vi "Test_Config.vi"() -> (3 "All Passed":bool)   [LabVIEW 2021]
uses:
  a98184f2-8fd2-43de-8bb4-98a66dcb5e40.vi
  80b57f80-8d76-4516-95c7-d8f010efd1e0.vi
  85257279-96b8-465d-b682-86ad9ca409f4.vi
  dc8dce16-54c7-48e3-a8d0-ee2a6ed5b8ba.vi
  b43f0ab9-3a27-4143-a30c-0508d2798f1e.vi
  76b3366a-3206-4512-a529-652fa6d884ac.vi
  2d5518fb-c5ca-40ab-9de5-64a59f6f1d1f.vi
  2ff284ed-e038-49b9-b7c6-f7e4ced53d45.vi
  80cedbcb-86fa-476a-b55d-adc21445b371.vi
  4e733a6e-a8c1-4522-8606-2b13abc68f21.vi
  2655c138-ab8e-4111-a2df-5fe2dfe4a7c9.vi
  41d25b3f-7330-49a0-a764-42fdbbcff171.vi
  f7d9e632-003d-414d-bfce-bb79d7acb7ab.vi
  0279d870-c547-41fe-a729-ccd6f17232ba.vi
  8ff58d8c-39b3-443f-854e-0b9261e8d6a6.vi
  70d4e39b-dee4-4ea3-9cfd-b708fc97263a.vi
  a490dff2-e7e9-4792-baf0-702021434066.vi
  e326765a-9b9c-4b66-87f7-89ea6da7ec42.vi
  c037a717-6626-4282-85e0-497ccd3c4725.vi
  bc476a8b-c6ff-4744-88c1-a1946416cf06.vi
  3efe5734-2677-4856-90c7-08a3cd52a3b4.vi
  b62ae4c1-b65b-4156-9e59-aa89f562b7c2.vi
  d670cadd-57b7-44dd-9da6-c55518de0625.vi
  e85abf48-7778-4a54-96b8-6050ae3c274e.vi
  56efa82e-35ee-46c5-92d5-02654ef11c94.vi
  dab66c0f-6c3b-4909-9241-b858b76ef6f7.vi
  747298a2-2a9b-49bf-9d1b-76691c951ae0.vi
  29b0d965-e3aa-4d7c-908d-78c0fd6e1640.vi
  d4e3c187-ed36-4e66-b6bb-bd3ba352b96f.vi
  83e091ec-0c56-40c0-b4cc-2b8daf4164db.vi
  3d9b7528-4a5f-4daa-a7a8-b912a6b1f25e.vi
  f850aa45-a057-498a-96bd-8df103c2ec00.vi
  04663b24-a35a-4e7f-83d2-43bb6f822b82.vi
  9bed9d14-1784-4e91-a23c-442c56fd1ce7.vi
  cdbf88fd-1480-460b-834e-4cc60c3bbcb4.vi
  src/SubVIs/Quotes.vi
  src/SubVIs/Key.vi
  <vilib>/Utility/error.llb/Error Cluster From Error Code.vi
  src/Config.lvlib
panel:
  out "Tests":cluster{"Test":string, "Passed":bool}[](array[cluster])
  out "Text":string
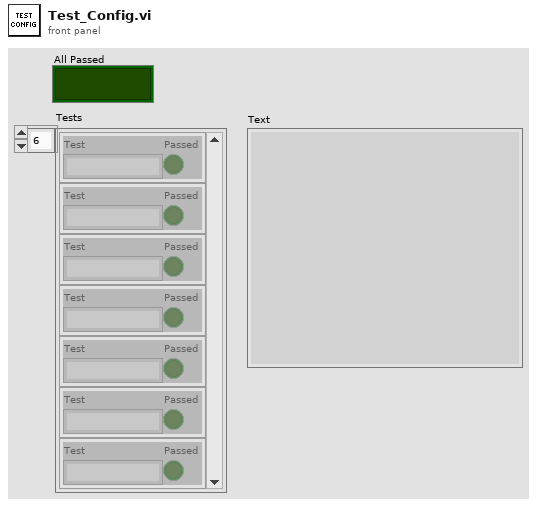
[diagram p1: front panel]
types:
  T1 = cluster{"Section":string, "Keys":cluster{"Key":string, "Value":string}[]}[]
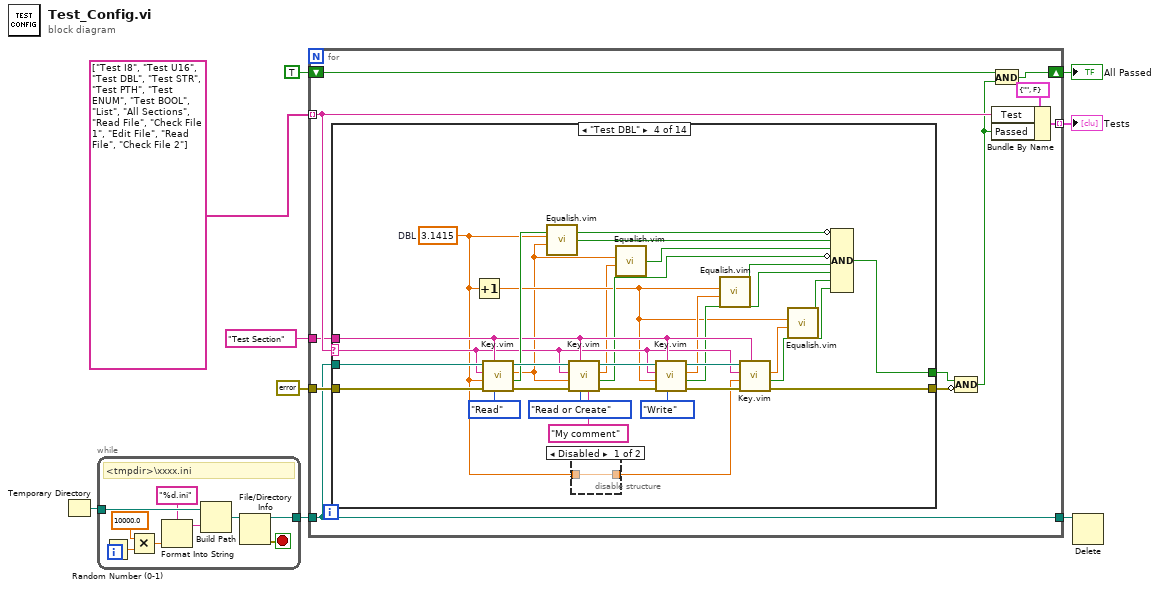
[diagram p0: block diagram]
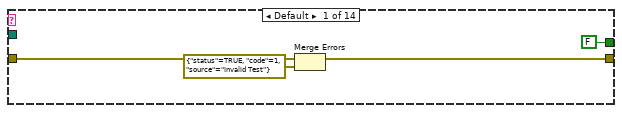
[diagram p2: hidden frame]
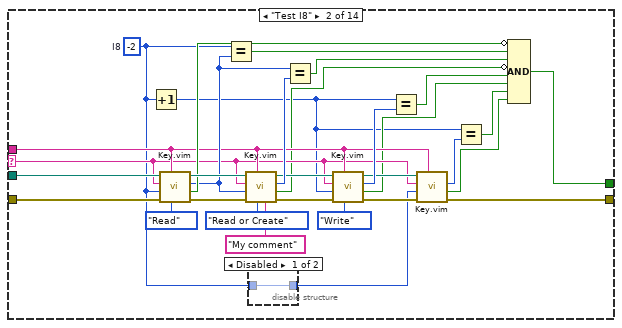
[diagram p3: hidden frame]
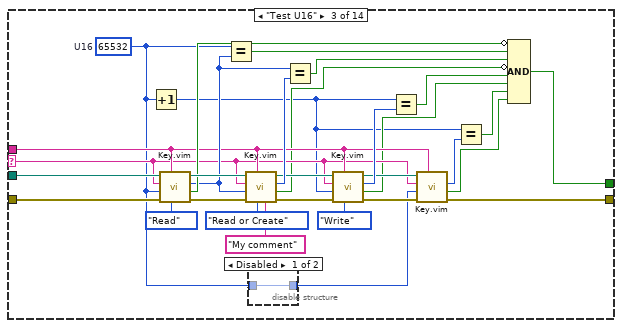
[diagram p5: hidden frame]
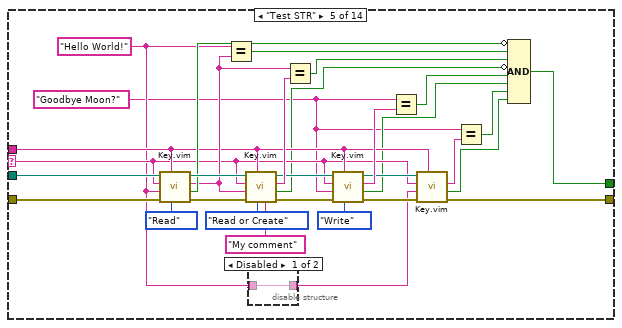
[diagram p8: hidden frame]
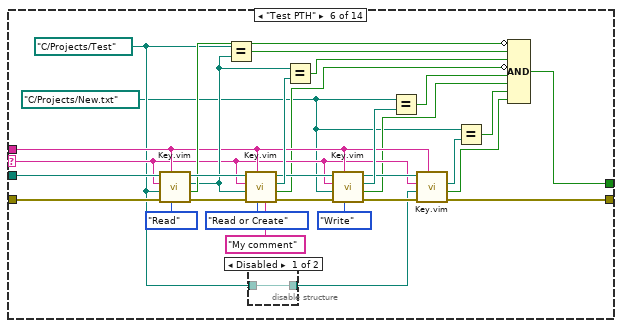
[diagram p10: hidden frame]
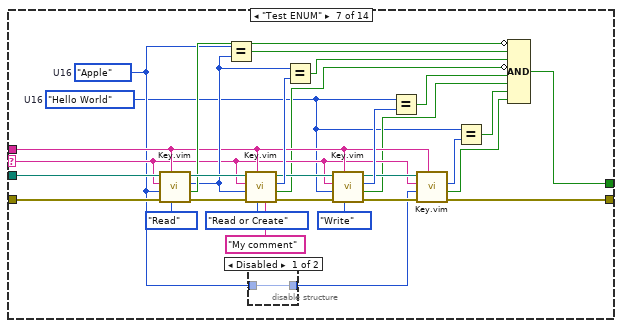
[diagram p12: hidden frame]
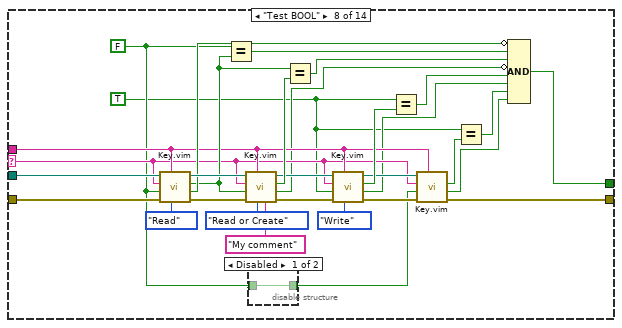
[diagram p14: hidden frame]
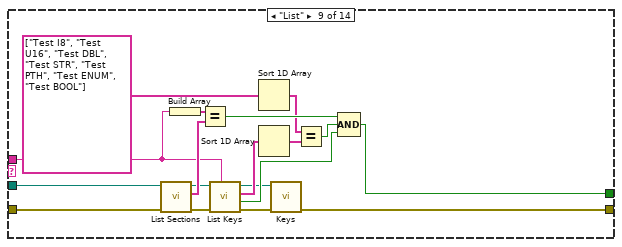
[diagram p16: hidden frame]
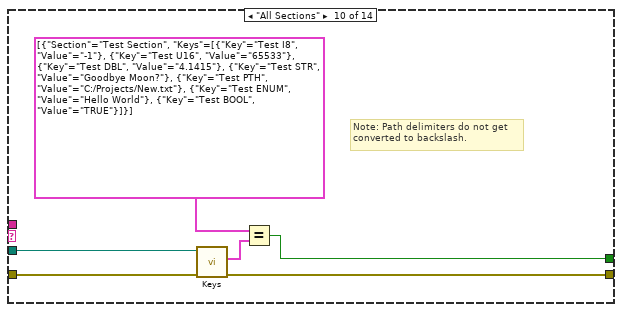
[diagram p17: hidden frame]
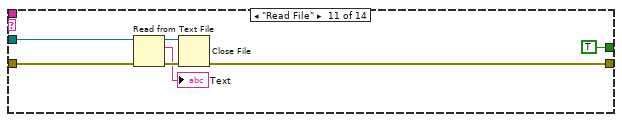
[diagram p18: hidden frame]
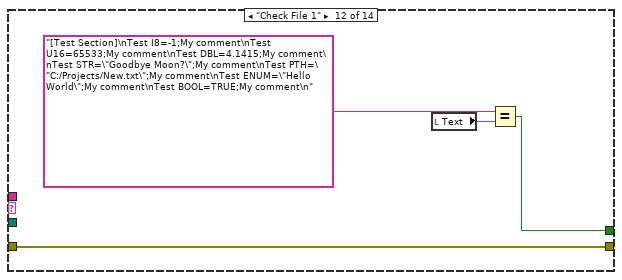
[diagram p19: hidden frame]
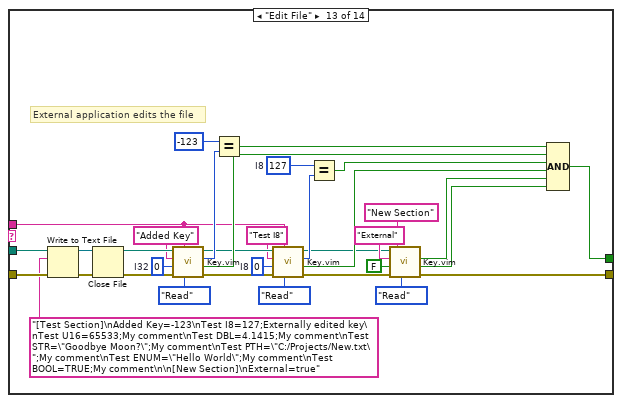
[diagram p20: hidden frame]
diagram:
  n1 = Temporary Directory() -> (w9:path)
  n2 = while {
    tunnel: w9 -> [w18]
    tunnel: [w10] -> w8
    stop <- w11 stop-if-true
    # "<tmpdir>\\xxxx.ini"
    n3 = Random Number (0-1)() -> (number: 0 to 1=w17:dbl)
    n4 = Multiply(x=10000.0 ("y"), y=w17) -> (x*y=w16:dbl)
    n5 = Format Into String(format string="%d.ini", w16) -> (resulting string=w13:string)  [unwired: 2 in, 1 out]
    n6 = Build Path(base path=w18, name or relative path=w13) -> (appended path=w12:path)
    n7 = File/Directory Info(path=w12) -> (path out=w10:path, error out=w11:errorcluster)  [unwired: 1 in, 5 out]
  }
  n8 = for {
    tunnel: w8 -> [w28]
    tunnel: errorcluster {"status"=FALSE, "code"=0, "source"=""} ("error out") -> [w29]
    tunnel: [w28] -> w6
    tunnel: string[] ["Test I8", "Test U16", "Test DBL", "Test STR", "Test PTH", "Test ENUM", "Test BOOL", "List", "All Sections", "Read File", "Check File 1", "Edit File", "Read File", "Check File 2"] ("array") -> [w24] mode=indexing
    tunnel: [w26] -> w5 mode=indexing
    shift-right: [w21] -> w2
    shift-left: TRUE -> [w22]
    tunnel: "Test Section" ("Section") -> [w19]
    n9 = case shown="\"Test DBL\"" w24 {
      selector: w24 -> [_ w44 w76 w114 w140 w172 w204 w236 _ _ _ _ _ _]
      tunnel: w29 -> [w33 w64 w96 w128 w160 w192 w224 w256 w275 w280 w286 w290 w324 w329]
      tunnel: w28 -> [_ w62 w94 w126 w158 w190 w222 w254 w274 w279 w285 _ w323 _]
      tunnel: [w32 w39 w71 w110 w135 w167 w200 w232 w260 w281 w284 w290 w293 w329] -> w23
      tunnel: w19 -> [_ w45 w77 w115 w141 w173 w205 w237 w269 _ _ _ w309 _]
      tunnel: [FALSE w34 w66 w108 w131 w163 w196 w228 w264 w277 TRUE w291 w306 w330] -> w25
      frame Default {
        n10 = Merge Errors(w33, errorcluster {"status"=TRUE, "code"=1, "source"="Invalid Test"} ("error in")) -> (w32:errorcluster)
      }
      frame "Test I8" {
        w40 = i8 -2  # I8
        n11 = Increment(x=w40) -> (x+1=w38:i8)
        n12 = call "Key.vim"("Operation (Read or Create)"=enum8{"Read or Create", "Read", "Write"}."Read", "Section"=w45, "error in (no error)"=w64, "Value"=w40, "Key"=w44, "Ini Path in"=w62) -> ("error out"=w60:errorcluster, "Found?"=w57:bool, "Value out"=w56:i8, "Ini Path out"=w59:path)  [unwired: 2 in]
        n13 = Equal?(x=w40, y=w56) -> (x = y?=w58:bool)
        n14 = call "Key.vim"("Comment (Create only)"="My comment", "Operation (Read or Create)"=enum8{"Read or Create", "Read", "Write"}."Read or Create", "Section"=w45, "error in (no error)"=w60, "Value"=w56, "Key"=w44, "Ini Path in"=w59) -> ("error out"=w51:errorcluster, "Found?"=w42:bool, "Value out"=w55:i8, "Ini Path out"=w50:path)  [unwired: 1 in]
        n15 = disable-structure shown="Disabled" {
          disable-tunnel: [w65 _] -> w41
          disable-tunnel: w40 -> [w65 _]
          frame Disabled {
          }
          frame Enabled {
          }
        }
        n16 = Equal?(x=w56, y=w55) -> (x = y?=w54:bool)
        n17 = call "Key.vim"("Operation (Read or Create)"=enum8{"Read or Create", "Read", "Write"}."Write", "Section"=w45, "error in (no error)"=w51, "Value"=w38, "Key"=w44, "Ini Path in"=w50) -> ("error out"=w47:errorcluster, "Found?"=w43:bool, "Value out"=w49:i8, "Ini Path out"=w46:path)  [unwired: 2 in]
        n18 = Equal?(x=w38, y=w49) -> (x = y?=w48:bool)
        n19 = call "Key.vim"("Section"=w45, "error in (no error)"=w47, "Value"=w41, "Key"=w44, "Ini Path in"=w46) -> ("error out"=w39:errorcluster, "Found?"=w35:bool, "Value out"=w37:i8)  [unwired: 3 in, 1 out]
        n20 = Equal?(x=w38, y=w37) -> (x = y?=w36:bool)
        n21 = Compound Arithmetic op=AND(invert w57, w58, w54, invert w42, w48, w43, w36, w35) -> (w34:bool)
      }
      frame "Test U16" {
        w72 = u16 65532  # U16
        n22 = Increment(x=w72) -> (x+1=w70:u16)
        n23 = call "Key.vim"("Operation (Read or Create)"=enum8{"Read or Create", "Read", "Write"}."Read", "Section"=w77, "error in (no error)"=w96, "Value"=w72, "Key"=w76, "Ini Path in"=w94) -> ("error out"=w92:errorcluster, "Found?"=w89:bool, "Value out"=w88:u16, "Ini Path out"=w91:path)  [unwired: 2 in]
        n24 = Equal?(x=w72, y=w88) -> (x = y?=w90:bool)
        n25 = call "Key.vim"("Comment (Create only)"="My comment", "Operation (Read or Create)"=enum8{"Read or Create", "Read", "Write"}."Read or Create", "Section"=w77, "error in (no error)"=w92, "Value"=w88, "Key"=w76, "Ini Path in"=w91) -> ("error out"=w83:errorcluster, "Found?"=w74:bool, "Value out"=w87:u16, "Ini Path out"=w82:path)  [unwired: 1 in]
        n26 = disable-structure shown="Disabled" {
          disable-tunnel: [w97 _] -> w73
          disable-tunnel: w72 -> [w97 _]
          frame Disabled {
          }
          frame Enabled {
          }
        }
        n27 = Equal?(x=w88, y=w87) -> (x = y?=w86:bool)
        n28 = call "Key.vim"("Operation (Read or Create)"=enum8{"Read or Create", "Read", "Write"}."Write", "Section"=w77, "error in (no error)"=w83, "Value"=w70, "Key"=w76, "Ini Path in"=w82) -> ("error out"=w79:errorcluster, "Found?"=w75:bool, "Value out"=w81:u16, "Ini Path out"=w78:path)  [unwired: 2 in]
        n29 = Equal?(x=w70, y=w81) -> (x = y?=w80:bool)
        n30 = call "Key.vim"("Section"=w77, "error in (no error)"=w79, "Value"=w73, "Key"=w76, "Ini Path in"=w78) -> ("error out"=w71:errorcluster, "Found?"=w67:bool, "Value out"=w69:u16)  [unwired: 3 in, 1 out]
        n31 = Equal?(x=w70, y=w69) -> (x = y?=w68:bool)
        n32 = Compound Arithmetic op=AND(invert w89, w90, w86, invert w74, w80, w75, w68, w67) -> (w66:bool)
      }
      frame "Test DBL" {
        w102 = 3.1415  # DBL
        n33 = Increment(x=w102) -> (x+1=w105:dbl)
        n34 = call "Key.vim"("Operation (Read or Create)"=enum8{"Read or Create", "Read", "Write"}."Read", "Section"=w115, "error in (no error)"=w128, "Value"=w102, "Key"=w114, "Ini Path in"=w126) -> ("error out"=w124:errorcluster, "Found?"=w122:bool, "Value out"=w100:dbl, "Ini Path out"=w123:path)  [unwired: 2 in]
        n35 = call "Equalish.vim"("First"=w102, "Second"=w100) -> ("Equal?"=w101:bool)  [unwired: 3 in]
        n36 = call "Key.vim"("Comment (Create only)"="My comment", "Operation (Read or Create)"=enum8{"Read or Create", "Read", "Write"}."Read or Create", "Section"=w115, "error in (no error)"=w124, "Value"=w100, "Key"=w114, "Ini Path in"=w123) -> ("error out"=w119:errorcluster, "Found?"=w112:bool, "Value out"=w99:dbl, "Ini Path out"=w118:path)  [unwired: 1 in]
        n37 = disable-structure shown="Disabled" {
          disable-tunnel: [w129 _] -> w111
          disable-tunnel: w102 -> [w129 _]
          frame Disabled {
          }
          frame Enabled {
          }
        }
        n38 = call "Equalish.vim"("First"=w100, "Second"=w99) -> ("Equal?"=w98:bool)  [unwired: 3 in]
        n39 = call "Key.vim"("Operation (Read or Create)"=enum8{"Read or Create", "Read", "Write"}."Write", "Section"=w115, "error in (no error)"=w119, "Value"=w105, "Key"=w114, "Ini Path in"=w118) -> ("error out"=w117:errorcluster, "Found?"=w113:bool, "Value out"=w107:dbl, "Ini Path out"=w116:path)  [unwired: 2 in]
        n40 = call "Equalish.vim"("First"=w105, "Second"=w107) -> ("Equal?"=w106:bool)  [unwired: 3 in]
        n41 = call "Key.vim"("Section"=w115, "error in (no error)"=w117, "Value"=w111, "Key"=w114, "Ini Path in"=w116) -> ("error out"=w110:errorcluster, "Found?"=w109:bool, "Value out"=w104:dbl)  [unwired: 3 in, 1 out]
        n42 = call "Equalish.vim"("First"=w105, "Second"=w104) -> ("Equal?"=w103:bool)  [unwired: 3 in]
        n43 = Compound Arithmetic op=AND(invert w122, w101, w98, invert w112, w106, w113, w103, w109) -> (w108:bool)
      }
      frame "Test STR" {
        w130 = "Goodbye Moon?"
        w136 = "Hello World!"
        n44 = call "Key.vim"("Operation (Read or Create)"=enum8{"Read or Create", "Read", "Write"}."Read", "Section"=w141, "error in (no error)"=w160, "Value"=w136, "Key"=w140, "Ini Path in"=w158) -> ("error out"=w156:errorcluster, "Found?"=w153:bool, "Value out"=w152:string, "Ini Path out"=w155:path)  [unwired: 2 in]
        n45 = Equal?(x=w136, y=w152) -> (x = y?=w154:bool)
        n46 = call "Key.vim"("Comment (Create only)"="My comment", "Operation (Read or Create)"=enum8{"Read or Create", "Read", "Write"}."Read or Create", "Section"=w141, "error in (no error)"=w156, "Value"=w152, "Key"=w140, "Ini Path in"=w155) -> ("error out"=w147:errorcluster, "Found?"=w138:bool, "Value out"=w151:string, "Ini Path out"=w146:path)  [unwired: 1 in]
        n47 = disable-structure shown="Disabled" {
          disable-tunnel: [w161 _] -> w137
          disable-tunnel: w136 -> [w161 _]
          frame Disabled {
          }
          frame Enabled {
          }
        }
        n48 = Equal?(x=w152, y=w151) -> (x = y?=w150:bool)
        n49 = call "Key.vim"("Operation (Read or Create)"=enum8{"Read or Create", "Read", "Write"}."Write", "Section"=w141, "error in (no error)"=w147, "Value"=w130, "Key"=w140, "Ini Path in"=w146) -> ("error out"=w143:errorcluster, "Found?"=w139:bool, "Value out"=w145:string, "Ini Path out"=w142:path)  [unwired: 2 in]
        n50 = Equal?(x=w130, y=w145) -> (x = y?=w144:bool)
        n51 = call "Key.vim"("Section"=w141, "error in (no error)"=w143, "Value"=w137, "Key"=w140, "Ini Path in"=w142) -> ("error out"=w135:errorcluster, "Found?"=w132:bool, "Value out"=w134:string)  [unwired: 3 in, 1 out]
        n52 = Equal?(x=w130, y=w134) -> (x = y?=w133:bool)
        n53 = Compound Arithmetic op=AND(invert w153, w154, w150, invert w138, w144, w139, w133, w132) -> (w131:bool)
      }
      frame "Test PTH" {
        w162 = path "C:/Projects/New.txt"
        w168 = path "C:/Projects/Test"
        n54 = call "Key.vim"("Operation (Read or Create)"=enum8{"Read or Create", "Read", "Write"}."Read", "Section"=w173, "error in (no error)"=w192, "Value"=w168, "Key"=w172, "Ini Path in"=w190) -> ("error out"=w188:errorcluster, "Found?"=w185:bool, "Value out"=w184:path, "Ini Path out"=w187:path)  [unwired: 2 in]
        n55 = Equal?(x=w168, y=w184) -> (x = y?=w186:bool)
        n56 = call "Key.vim"("Comment (Create only)"="My comment", "Operation (Read or Create)"=enum8{"Read or Create", "Read", "Write"}."Read or Create", "Section"=w173, "error in (no error)"=w188, "Value"=w184, "Key"=w172, "Ini Path in"=w187) -> ("error out"=w179:errorcluster, "Found?"=w170:bool, "Value out"=w183:path, "Ini Path out"=w178:path)  [unwired: 1 in]
        n57 = disable-structure shown="Disabled" {
          disable-tunnel: [w193 _] -> w169
          disable-tunnel: w168 -> [w193 _]
          frame Disabled {
          }
          frame Enabled {
          }
        }
        n58 = Equal?(x=w184, y=w183) -> (x = y?=w182:bool)
        n59 = call "Key.vim"("Operation (Read or Create)"=enum8{"Read or Create", "Read", "Write"}."Write", "Section"=w173, "error in (no error)"=w179, "Value"=w162, "Key"=w172, "Ini Path in"=w178) -> ("error out"=w175:errorcluster, "Found?"=w171:bool, "Value out"=w177:path, "Ini Path out"=w174:path)  [unwired: 2 in]
        n60 = Equal?(x=w162, y=w177) -> (x = y?=w176:bool)
        n61 = call "Key.vim"("Section"=w173, "error in (no error)"=w175, "Value"=w169, "Key"=w172, "Ini Path in"=w174) -> ("error out"=w167:errorcluster, "Found?"=w164:bool, "Value out"=w166:path)  [unwired: 3 in, 1 out]
        n62 = Equal?(x=w162, y=w166) -> (x = y?=w165:bool)
        n63 = Compound Arithmetic op=AND(invert w185, w186, w182, invert w170, w176, w171, w165, w164) -> (w163:bool)
      }
      frame "Test ENUM" {
        w194 = enum16{"Apple", "Hello World", "Item 3"}."Hello World"  # U16
        w195 = enum16{"Apple", "Hello World", "Item 3"}."Apple"  # U16
        n64 = call "Key.vim"("Operation (Read or Create)"=enum8{"Read or Create", "Read", "Write"}."Read", "Section"=w205, "error in (no error)"=w224, "Value"=w195, "Key"=w204, "Ini Path in"=w222) -> ("error out"=w220:errorcluster, "Found?"=w217:bool, "Value out"=w216:enum16{"Apple", "Hello World", "Item 3"}, "Ini Path out"=w219:path)  [unwired: 2 in]
        n65 = Equal?(x=w195, y=w216) -> (x = y?=w218:bool)
        n66 = call "Key.vim"("Comment (Create only)"="My comment", "Operation (Read or Create)"=enum8{"Read or Create", "Read", "Write"}."Read or Create", "Section"=w205, "error in (no error)"=w220, "Value"=w216, "Key"=w204, "Ini Path in"=w219) -> ("error out"=w211:errorcluster, "Found?"=w202:bool, "Value out"=w215:enum16{"Apple", "Hello World", "Item 3"}, "Ini Path out"=w210:path)  [unwired: 1 in]
        n67 = disable-structure shown="Disabled" {
          disable-tunnel: [w225 _] -> w201
          disable-tunnel: w195 -> [w225 _]
          frame Disabled {
          }
          frame Enabled {
          }
        }
        n68 = Equal?(x=w216, y=w215) -> (x = y?=w214:bool)
        n69 = call "Key.vim"("Operation (Read or Create)"=enum8{"Read or Create", "Read", "Write"}."Write", "Section"=w205, "error in (no error)"=w211, "Value"=w194, "Key"=w204, "Ini Path in"=w210) -> ("error out"=w207:errorcluster, "Found?"=w203:bool, "Value out"=w209:enum16{"Apple", "Hello World", "Item 3"}, "Ini Path out"=w206:path)  [unwired: 2 in]
        n70 = Equal?(x=w194, y=w209) -> (x = y?=w208:bool)
        n71 = call "Key.vim"("Section"=w205, "error in (no error)"=w207, "Value"=w201, "Key"=w204, "Ini Path in"=w206) -> ("error out"=w200:errorcluster, "Found?"=w197:bool, "Value out"=w199:enum16{"Apple", "Hello World", "Item 3"})  [unwired: 3 in, 1 out]
        n72 = Equal?(x=w194, y=w199) -> (x = y?=w198:bool)
        n73 = Compound Arithmetic op=AND(invert w217, w218, w214, invert w202, w208, w203, w198, w197) -> (w196:bool)
      }
      frame "Test BOOL" {
        w226 = TRUE
        w227 = FALSE
        n74 = call "Key.vim"("Operation (Read or Create)"=enum8{"Read or Create", "Read", "Write"}."Read", "Section"=w237, "error in (no error)"=w256, "Value"=w227, "Key"=w236, "Ini Path in"=w254) -> ("error out"=w252:errorcluster, "Found?"=w249:bool, "Value out"=w248:bool, "Ini Path out"=w251:path)  [unwired: 2 in]
        n75 = Equal?(x=w227, y=w248) -> (x = y?=w250:bool)
        n76 = call "Key.vim"("Comment (Create only)"="My comment", "Operation (Read or Create)"=enum8{"Read or Create", "Read", "Write"}."Read or Create", "Section"=w237, "error in (no error)"=w252, "Value"=w248, "Key"=w236, "Ini Path in"=w251) -> ("error out"=w243:errorcluster, "Found?"=w234:bool, "Value out"=w247:bool, "Ini Path out"=w242:path)  [unwired: 1 in]
        n77 = disable-structure shown="Disabled" {
          disable-tunnel: [w257 _] -> w233
          disable-tunnel: w227 -> [w257 _]
          frame Disabled {
          }
          frame Enabled {
          }
        }
        n78 = Equal?(x=w248, y=w247) -> (x = y?=w246:bool)
        n79 = call "Key.vim"("Operation (Read or Create)"=enum8{"Read or Create", "Read", "Write"}."Write", "Section"=w237, "error in (no error)"=w243, "Value"=w226, "Key"=w236, "Ini Path in"=w242) -> ("error out"=w239:errorcluster, "Found?"=w235:bool, "Value out"=w241:bool, "Ini Path out"=w238:path)  [unwired: 2 in]
        n80 = Equal?(x=w226, y=w241) -> (x = y?=w240:bool)
        n81 = call "Key.vim"("Section"=w237, "error in (no error)"=w239, "Value"=w233, "Key"=w236, "Ini Path in"=w238) -> ("error out"=w232:errorcluster, "Found?"=w229:bool, "Value out"=w231:bool)  [unwired: 3 in, 1 out]
        n82 = Equal?(x=w226, y=w231) -> (x = y?=w230:bool)
        n83 = Compound Arithmetic op=AND(invert w249, w250, w246, invert w234, w240, w235, w230, w229) -> (w228:bool)
      }
      frame "List" {
        n84 = call "List Sections.vi"("error in (no error)"=w275, "Ini Path in"=w274) -> ("error out"=w271:errorcluster, "Sections"=w273:string[], "Ini Path out"=w270:path)  [unwired: 7 in]
        n85 = Build Array(w269) -> (w272:string[])
        n86 = Equal?(x=w272, y=w273) -> (x = y?=w268:bool)
        n87 = call "List Keys.vi"("Section"=w269, "error in (no error)"=w271, "Ini Path in"=w270) -> ("error out"=w261:errorcluster, "Section Found?"=w262:bool, "Keys"=w267:string[], "Ini Path out"=w259:path)  [unwired: 5 in]
        n88 = Sort 1D Array(array=string[] ["Test I8", "Test U16", "Test DBL", "Test STR", "Test PTH", "Test ENUM", "Test BOOL"] ("Keys")) -> (sorted array=w263:string[])
        n89 = Sort 1D Array(array=w267) -> (sorted array=w266:string[])
        n90 = call "Keys.vi"("error in (no error)"=w261, "Ini Path in"=w259) -> ("error out"=w260:errorcluster)  [unwired: 7 in, 2 out]
        n91 = Equal?(x=w263, y=w266) -> (x = y?=w265:bool)
        n92 = Compound Arithmetic op=AND(w268, w265, w262) -> (w264:bool)
      }
      frame "All Sections" {
        # "Note: Path delimiters do not get\nconverted to backslash."
        n93 = call "Keys.vi"("error in (no error)"=w280, "Ini Path in"=w279) -> ("error out"=w281:errorcluster, "Sections"=w278:T1)  [unwired: 7 in, 1 out]
        n94 = Equal?(x=T1 [{"Section"="Test Section", "Keys"=[{"Key"="Test I8", "Value"="-1"}, {"Key"="Test U16", "Value"="65533"}, {"Key"="Test DBL", "Value"="4.1415"}, {"Key"="Test STR", "Value"="Goodbye Moon?"}, {"Key"="Test PTH", "Value"="C:/Projects/New.txt"}, {"Key"="Test ENUM", "Value"="Hello World"}, {"Key"="Test BOOL", "Value"="TRUE"}]}] ("Sections"), y=w278) -> (x = y?=w277:bool)
      }
      frame "Read File" {
        n95 = Read from Text File(file (use dialog)=w285, error in=w286) -> (refnum out=w288:refnum<file>, text=→"Text":string, error out=w287:errorcluster)  [unwired: 2 in, 1 out]
        n96 = Close File(refnum=w288, error in=w287) -> (error out=w284:errorcluster)  [unwired: 1 out]
      }
      frame "Check File 1" {
        n97 = local read "Text"() -> (w289:string)
        n98 = Equal?(x="[Test Section]\nTest I8=-1;My comment\nTest U16=65533;My comment\nTest DBL=4.1415;My comment\nTest STR=\"Goodbye Moon?\";My comment\nTest PTH=\"C:/Projects/New.txt\";My comment\nTest ENUM=\"Hello World\";My comment\nTest BOOL=TRUE;My comment\n" ("Text"), y=w289) -> (x = y?=w291:bool)
      }
      frame "Edit File" {
        w304 = i8 127  # I8
        w307 = i8 0  # I8
        w318 = 0  # I32
        # "External application edits the file"
        n99 = Write to Text File(file (use dialog)=w323, text="[Test Section]\nAdded Key=-123\nTest I8=127;Externally edited key\nTest U16=65533;My comment\nTest DBL=4.1415;My comment\nTest STR=\"Goodbye Moon?\";My comment\nTest PTH=\"C:/Projects/New.txt\";My comment\nTest ENUM=\"Hello World\";My comment\nTest BOOL=TRUE;My comment\n\n[New Section]\nExternal=true" ("Text"), error in=w324) -> (refnum out=w326:refnum<file>, error out=w325:errorcluster)  [unwired: 1 in, 1 out]
        n100 = Close File(refnum=w326, error in=w325) -> (path=w321:path, error out=w320:errorcluster)
        n101 = call "Key.vim"("Operation (Read or Create)"=enum8{"Read or Create", "Read", "Write"}."Read", "Section"=w309, "error in (no error)"=w320, "Value"=w318, "Key"="Added Key", "Ini Path in"=w321) -> ("error out"=w311:errorcluster, "Found?"=w313:bool, "Value out"=w316:i32, "Ini Path out"=w310:path)  [unwired: 2 in]
        n102 = Equal?(x=-123 ("y"), y=w316) -> (x = y?=w314:bool)
        n103 = call "Key.vim"("Operation (Read or Create)"=enum8{"Read or Create", "Read", "Write"}."Read", "Section"=w309, "error in (no error)"=w311, "Value"=w307, "Key"="Test I8", "Ini Path in"=w310) -> ("error out"=w298:errorcluster, "Found?"=w305:bool, "Value out"=w303:i8, "Ini Path out"=w297:path)  [unwired: 2 in]
        n104 = Equal?(x=w304, y=w303) -> (x = y?=w302:bool)
        n105 = call "Key.vim"("Operation (Read or Create)"=enum8{"Read or Create", "Read", "Write"}."Read", "Section"="New Section", "error in (no error)"=w298, "Value"=FALSE, "Key"="External", "Ini Path in"=w297) -> ("error out"=w293:errorcluster, "Found?"=w294:bool, "Value out"=w295:bool)  [unwired: 2 in, 1 out]
        n106 = Compound Arithmetic op=AND(w314, w313, w302, w305, w295, w294) -> (w306:bool)
      }
      frame "Check File 2" {
        n107 = local read "Text"() -> (w328:string)
        n108 = Equal?(x="[Test Section]\nAdded Key=-123\nTest I8=127;Externally edited key\nTest U16=65533;My comment\nTest DBL=4.1415;My comment\nTest STR=\"Goodbye Moon?\";My comment\nTest PTH=\"C:/Projects/New.txt\";My comment\nTest ENUM=\"Hello World\";My comment\nTest BOOL=TRUE;My comment\n\n[New Section]\nExternal=true" ("Text"), y=w328) -> (x = y?=w330:bool)
      }
    }
    n109 = Compound Arithmetic op=AND(w25, invert w23) -> (w20:bool)
    n110 = And(x=w22, y=w20) -> (x .and. y?=w21:bool)
    n111 = Bundle By Name(cluster=cluster{"Test":string, "Passed":bool} {"Test"="", "Passed"=FALSE} ("Cluster"), "Test"=w24, "Passed"=w20) -> (w26:cluster{"Test":string, "Passed":bool})
  }
  "Tests" <- w5
  "All Passed" <- w2
  n112 = Delete(path (use dialog)=w6) -> ()  [unwired: 4 in, 3 out]
